vi "Set-Background-correction.vi"(8 "error in (no error)":errorcluster, 10 "Correct. params in":refnum<data-value>, 11 "PF_MV1-D1312-240 in":refnum<class "PF_MV1-D1312-240.lvclass">) -> (0 "error out":errorcluster, 2 "Correct. params":refnum<data-value>, 3 "PF_MV1-D1312-240 out":refnum<class "PF_MV1-D1312-240.lvclass">)   [LabVIEW 2013, in "CameraVision.lvlib" / "PF_MV1-D1312-240.lvclass"]
uses:
  PF_MV1-D1312-240.lvclass
  Main/Correction/CV-Correction.lvclass
  Main/Correction/Background-correction.ctl
  Camera.lvclass/Camera.ctl
  Main/Correction/CV-Correction.lvclass/CV-Correction.ctl
  Main/Correction/Read Background correction.vi
  Main/Correction/Read Hotpixel correction.vi
  Main/Correction/Read Background correction type.vi
  <userlib>/Photonfocus Toolkit/_Public/SubVIs/pf_Set_Camera_Property_Mode.vi
  <userlib>/Photonfocus Toolkit/Photonfocus_Toolkit.lvlib
  Camera.lvclass
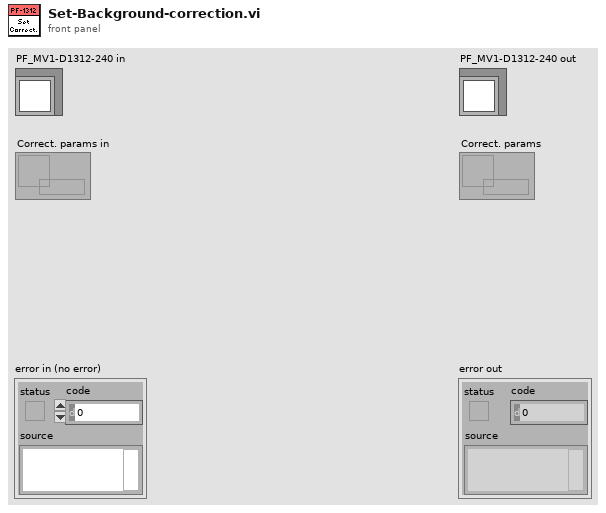
[diagram p1: front panel]
types:
  T1 = typedef "CameraVision.lvlib/CV-Correction.lvclass/Background-correction.ctl" = enum16{"Hardware", "Software"}
  T2 = typedef "CameraVision.lvlib/Correction.lvclass/Background-correction.ctl" = enum16{"Hardware", "Software"}
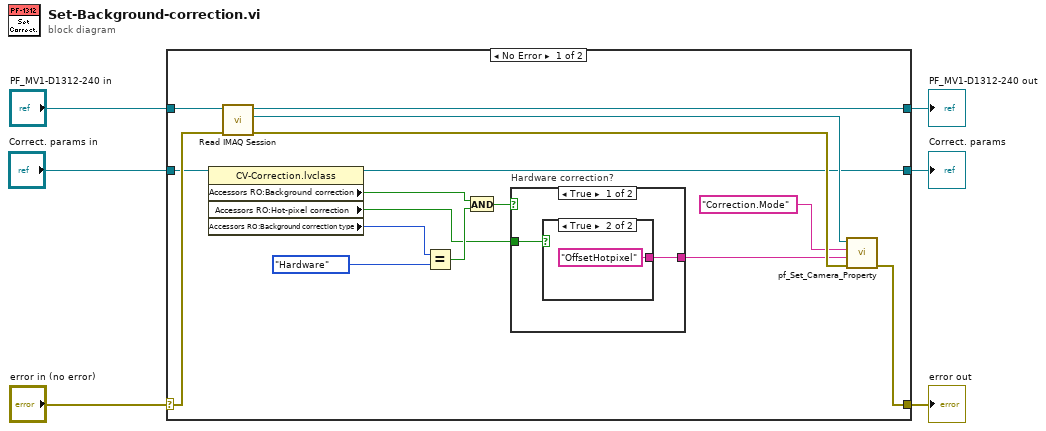
[diagram p0: block diagram]
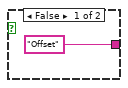
[diagram p2: hidden frame]
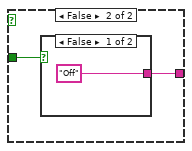
[diagram p3: hidden frame]
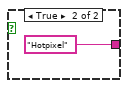
[diagram p4: hidden frame]
diagram:
  n1 = case shown="No Error" "error in (no error)" {
    selector: "error in (no error)" -> [w19 w33]
    tunnel: [w17 w33] -> w5
    tunnel: [w20 w32] -> w3
    tunnel: "PF_MV1-D1312-240 in" -> [w21 w32]
    tunnel: "Correct. params in" -> [w12 w31]
    tunnel: [w7 w31] -> w1
    frame No Error {
      n2 = property class="CV-Correction.lvclass"(reference=w12) -> (reference out=w7:refnum<data-value>, "Accessors RO:Background correction"=w9:bool, "Accessors RO:Hot-pixel correction"=w8:bool, "Accessors RO:Background correction type"=w10:T2)  [unwired: 1 in, 1 out]
      n3 = call "Read IMAQ Session.vi"("error in (no error)"=w19, "Camera in"=w21) -> ("error out"=w18:errorcluster, "IMAQ Session"=w22:refnum<k11>, "Camera out"=w20:refnum<class "PF_MV1-D1312-240.lvclass">)  [unwired: 7 in]
      n4 = Equal?(x=w10, y=Background-correction."Hardware" ("Background correction type")) -> (x = y?=w14:bool)
      n5 = And(x=w9, y=w14) -> (x .and. y?=w13:bool)
      n6 = case "Hardware correction?" shown="True" w13 {
        tunnel: [w24 w28] -> w15
        tunnel: w8 -> [w23 w27]
        frame True {
          n7 = case shown="True" w23 {
            tunnel: ["Offset" "OffsetHotpixel"] -> w24
            frame False {
            }
            frame True {
            }
          }
        }
        frame False {
          n8 = case shown="False" w27 {
            tunnel: ["Off" "Hotpixel"] -> w28
            frame False {
            }
            frame True {
            }
          }
        }
      }
      n9 = call-poly <userlib>:"pf_Set_Camera_Property.vi"("error in (no error)"=w18, "Property Value"=w15, "Property Name"="Correction.Mode", "IMAQ Session in"=w22) -> ("error out"=w17:errorcluster)  [unwired: 5 in, 2 out]
    }
    frame Error {
    }
  }
  "error out" <- w5
  "PF_MV1-D1312-240 out" <- w3
  "Correct. params" <- w1
